vi "Updata Current Sense Resistance List.vi"(11 "Array in":dbl[](array[numeric])) -> (3 "Array out":string[](array[string]))   [LabVIEW 2023]
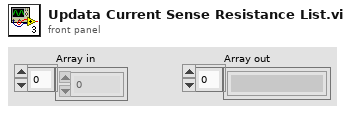
[diagram p1: front panel]
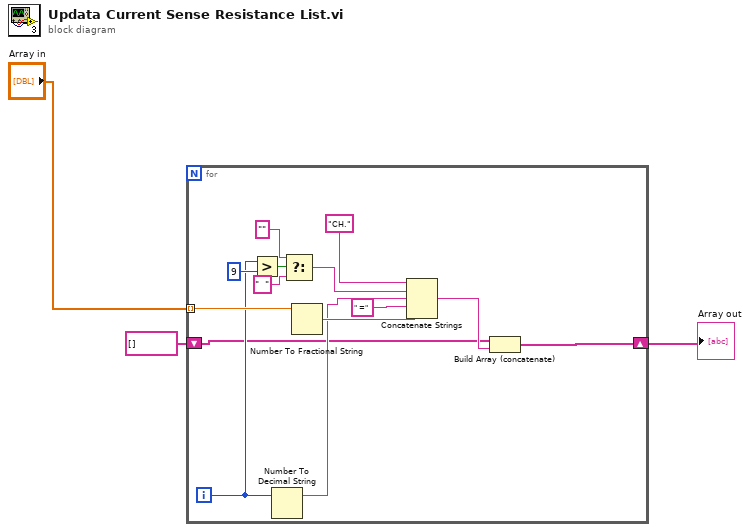
[diagram p0: block diagram]
diagram:
  n1 = for {
    tunnel: "Array in" -> [w8] mode=indexing
    shift-right: [w4] -> w3
    shift-left: string[] [] -> [w5]
    i -> [w7]
    n2 = Greater?(x=w7, y=9) -> (0:w12:bool)
    n3 = Number To Decimal String(number=w7) -> (decimal integer string=w16:string)  [unwired: 1 in]
    n4 = Select(t="" ("string"), s=w12, f="  " ("string")) -> (s? t:f=w11:string)
    n5 = Number To Fractional String(number=w8) -> (F-format string=w17:string)  [unwired: 3 in]
    n6 = Concatenate Strings("CH." ("string"), w11, w16, " =" ("string"), w17) -> (w6:string)
    n7 = Build Array (concatenate)(w5, w6) -> (w4:string[])
  }
  "Array out" <- w3
